vi "Main.vi"(0 "ActionsOnEvents in":refnum<class "ActionsOnEvents.lvclass">, 5 "error in (no error)":errorcluster) -> (14 "ActionsOnEvents out":refnum<class "ActionsOnEvents.lvclass">, 19 "error out":errorcluster)   [LabVIEW 2017, in "ActionsOnEvents.lvclass"]
uses:
  ActionsOnEvents.lvclass
  ActionsOnEvents.lvclass/ActionsOnEvents.ctl
  Actions/ActionBase_class/ActionBase.lvclass
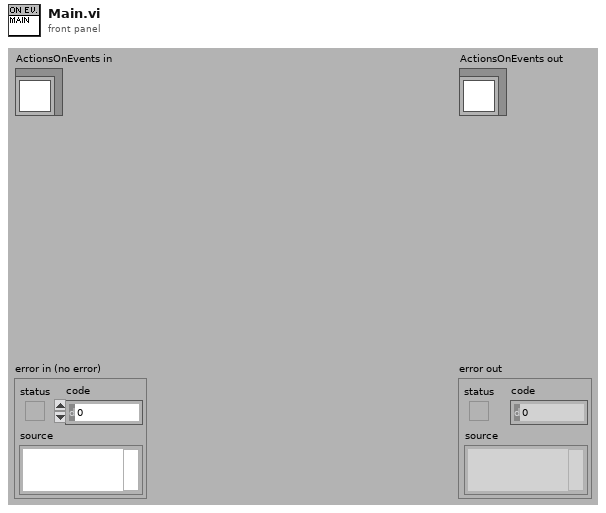
[diagram p1: front panel]
types:
  T1 = typedef "SystemEventsType.ctl" = cluster{"TrigOn":refnum<user-event>, "TrigOff":refnum<user-event>, "Result":refnum<user-event>, "Enable":refnum<user-event>, "Stop":refnum<user-event>, "AnalysisCompleted":refnum<user-event>, "Info":refnum<user-event>}
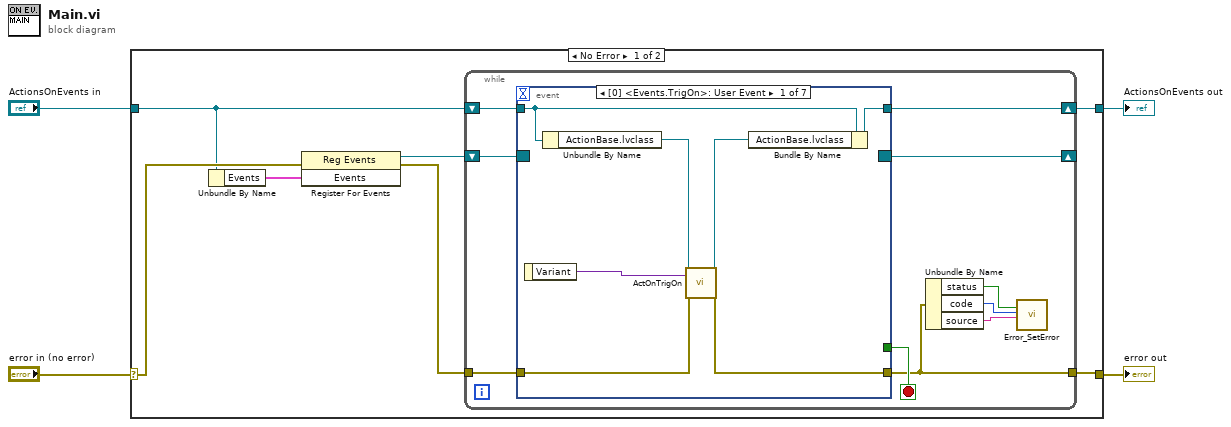
[diagram p0: block diagram]
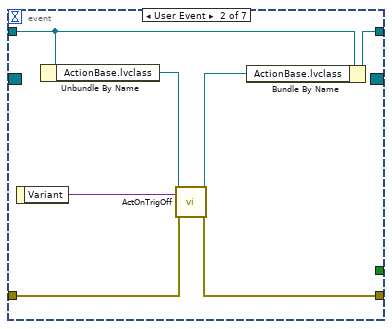
[diagram p2: hidden frame]
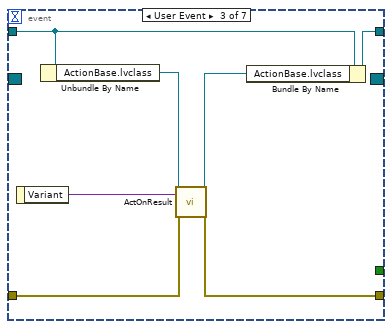
[diagram p3: hidden frame]
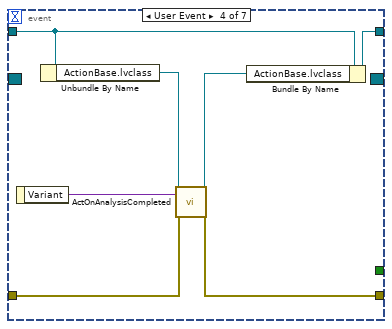
[diagram p4: hidden frame]
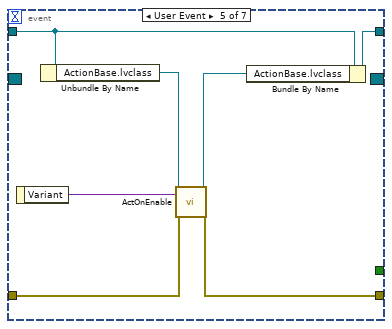
[diagram p5: hidden frame]
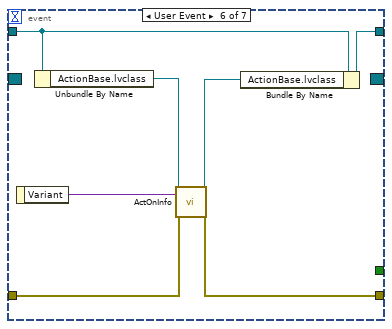
[diagram p6: hidden frame]
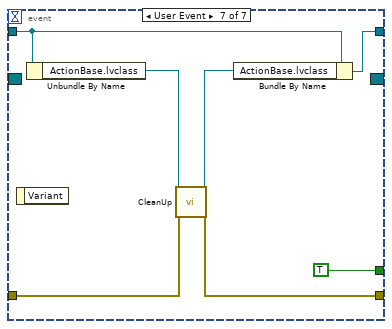
[diagram p7: hidden frame]
diagram:
  n1 = case shown="No Error" "error in (no error)" {
    selector: "error in (no error)" -> [w9 w72]
    tunnel: [w11 w72] -> w3
    tunnel: [w5 w71] -> w1
    tunnel: "ActionsOnEvents in" -> [w6 w71]
    frame No Error {
      n2 = Unbundle By Name(w6) -> ("Events"=w10:T1)
      n3 = register-events(error in=w9, w10) -> (reference out=w7:refnum<event-registration>, error out=w8:errorcluster)  [unwired: 1 in]
      n4 = while {
        shift-right: [w20] -> _
        shift-left: w7 -> [w21]
        shift-right: [w17] -> w5
        shift-left: w6 -> [w19]
        tunnel: w8 -> [w18]
        tunnel: [w13] -> w11
        stop <- w16 stop-if-true
        n5 = event shown="[0] <Events.TrigOn>: User Event" {
          selector: w21 -> [_ _ _ _ _ _ _]
          dyn-events: [_ _ _ _ _ _ _] -> w20
          timeout: _ -> [_ _ _ _ _ _ _]
          tunnel: w19 -> [w24 w32 w42 w49 w56 w63 w65]
          tunnel: w18 -> [w27 w35 w40 w47 w53 w59 w69]
          tunnel: [w26 w34 w36 w46 w52 w58 w68] -> w13
          tunnel: [w23 w30 w41 w48 w55 w62 w64] -> w17
          tunnel: [_ _ _ _ _ _ TRUE] -> w16
          event User Event {
            n6 = event-data() -> ("Variant"=w25:variant)  [unwired: 1 out]
            n7 = Unbundle By Name(w24) -> ("ActionBase.lvclass"=w28:refnum<class "ActionBase.lvclass">)
            n8 = call-dynamic "ActOnTrigOn.vi"("ActionBase in"=w28, "Data"=w25, "error in (no error)"=w27) -> ("ActionBase out"=w22:refnum<class "ActionBase.lvclass">, "error out"=w26:errorcluster)  [unwired: 15 out]
            n9 = Bundle By Name(cluster=w24, "ActionBase.lvclass"=w22) -> (w23:refnum<class "ActionsOnEvents.lvclass">)
          }
          event User Event {
            n10 = event-data() -> ("Variant"=w33:variant)  [unwired: 1 out]
            n11 = Unbundle By Name(w32) -> ("ActionBase.lvclass"=w31:refnum<class "ActionBase.lvclass">)
            n12 = call-dynamic "ActOnTrigOff.vi"("ActionBase in"=w31, "Data"=w33, "error in (no error)"=w35) -> ("ActionBase out"=w29:refnum<class "ActionBase.lvclass">, "error out"=w34:errorcluster)  [unwired: 15 out]
            n13 = Bundle By Name(cluster=w32, "ActionBase.lvclass"=w29) -> (w30:refnum<class "ActionsOnEvents.lvclass">)
          }
          event User Event {
            n14 = event-data() -> ("Variant"=w39:variant)  [unwired: 1 out]
            n15 = Unbundle By Name(w42) -> ("ActionBase.lvclass"=w38:refnum<class "ActionBase.lvclass">)
            n16 = call-dynamic "ActOnResult.vi"("ActionBase in"=w38, "Data"=w39, "error in (no error)"=w40) -> ("ActionBase out"=w37:refnum<class "ActionBase.lvclass">, "error out"=w36:errorcluster)  [unwired: 15 out]
            n17 = Bundle By Name(cluster=w42, "ActionBase.lvclass"=w37) -> (w41:refnum<class "ActionsOnEvents.lvclass">)
          }
          event User Event {
            n18 = event-data() -> ("Variant"=w45:variant)  [unwired: 1 out]
            n19 = Unbundle By Name(w49) -> ("ActionBase.lvclass"=w44:refnum<class "ActionBase.lvclass">)
            n20 = call-dynamic "ActOnAnalysisCompleted.vi"("ActionBase in"=w44, "Data"=w45, "error in (no error)"=w47) -> ("ActionBase out"=w43:refnum<class "ActionBase.lvclass">, "error out"=w46:errorcluster)  [unwired: 15 out]
            n21 = Bundle By Name(cluster=w49, "ActionBase.lvclass"=w43) -> (w48:refnum<class "ActionsOnEvents.lvclass">)
          }
          event User Event {
            n22 = event-data() -> ("Variant"=w54:variant)  [unwired: 1 out]
            n23 = Unbundle By Name(w56) -> ("ActionBase.lvclass"=w51:refnum<class "ActionBase.lvclass">)
            n24 = call-dynamic "ActOnEnable.vi"("ActionBase in"=w51, "Data"=w54, "error in (no error)"=w53) -> ("ActionBase out"=w50:refnum<class "ActionBase.lvclass">, "error out"=w52:errorcluster)  [unwired: 15 out]
            n25 = Bundle By Name(cluster=w56, "ActionBase.lvclass"=w50) -> (w55:refnum<class "ActionsOnEvents.lvclass">)
          }
          event User Event {
            n26 = event-data() -> ("Variant"=w57:variant)  [unwired: 1 out]
            n27 = Unbundle By Name(w63) -> ("ActionBase.lvclass"=w61:refnum<class "ActionBase.lvclass">)
            n28 = call-dynamic "ActOnInfo.vi"("ActionBase in"=w61, "Data"=w57, "error in (no error)"=w59) -> ("ActionBase out"=w60:refnum<class "ActionBase.lvclass">, "error out"=w58:errorcluster)  [unwired: 15 in]
            n29 = Bundle By Name(cluster=w63, "ActionBase.lvclass"=w60) -> (w62:refnum<class "ActionsOnEvents.lvclass">)
          }
          event User Event {
            n30 = event-data() -> ()  [unwired: 2 out]
            n31 = Unbundle By Name(w65) -> ("ActionBase.lvclass"=w67:refnum<class "ActionBase.lvclass">)
            n32 = call-dynamic "CleanUp.vi"("ActionBase in"=w67, "error in (no error)"=w69) -> ("ActionBase out"=w66:refnum<class "ActionBase.lvclass">, "error out"=w68:errorcluster)  [unwired: 16 out]
            n33 = Bundle By Name(cluster=w65, "ActionBase.lvclass"=w66) -> (w64:refnum<class "ActionsOnEvents.lvclass">)
          }
        }
        n34 = Unbundle By Name(w13) -> ("status"=w12:bool, "code"=w14:i32, "source"=w15:string)
        n35 = call "Error_SetError.vi"("status"=w12, "code (5000)"=w14, "source"=w15) -> ()  [unwired: 2 in, 15 out]
      }
    }
    frame Error {
    }
  }
  "error out" <- w3
  "ActionsOnEvents out" <- w1
